vi "test harness_FXP_A_times_x_iterate.vi"() -> ()   [LabVIEW 2017, in "FXP_observer_TestCase.lvclass"]
uses:
  FXP_observer_TestCase.lvclass
  fpga_VIs/fixed-point/typeDefs/x_vec_scalar.ctl
  <vilib>/rvi/DesktopExecutionNode/Execution/niFpgaDEN_Execute.vi
  <vilib>/rvi/DesktopExecutionNode/DesktopExecutionNode.xnode
panel:
  out "X_vec":T1[](array[typedef])
  out "xk_1_1":fxp<+/-,32,6>[](array[numeric])
  out "A*x":fxp<+/-,32,13>[](array[numeric])
  out "y(exp)":fxp<+/-,64,17>
  out "A*x (expected)":fxp<+/-,64,12>[](array[numeric])
  out "Waveform Graph":dbl[](graph)
  out "Y":fxp<+/-,32,6>[](array[numeric])
  in  "NumIter":i32
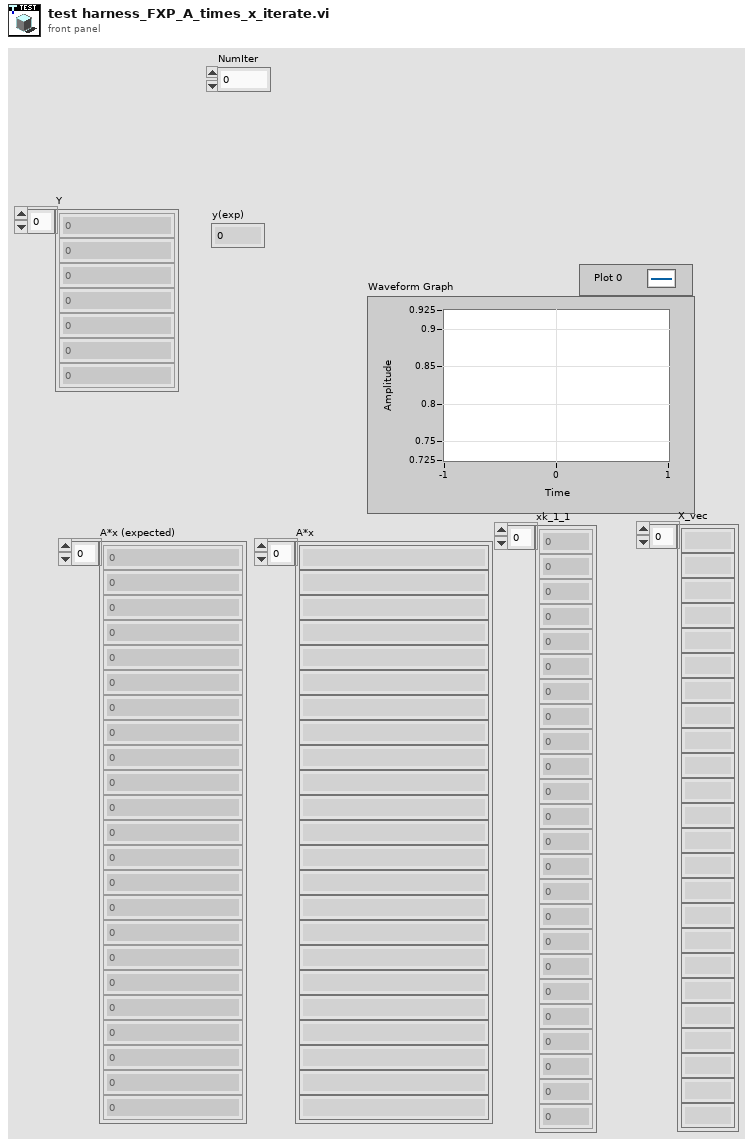
[diagram p1: front panel]
types:
  T1 = typedef "x_vec_scalar.ctl" = fxp<+/-,32,6>
  T2 = typedef "UT_matrix_data.ctl" = cluster{"Bz":T3[], "Ldist":T4[], "Kz":T5[], "Nx":T6[], "Ax_col":T7[], "X_vec":T1[], "Cz":T8[]}
  T3 = typedef "Bz_vec_scalar.ctl" = fxp<+/-,32,3>
  T4 = typedef "Lz_vec_scalar.ctl" = fxp<+/-,32,3>
  T5 = typedef "Kz_vec_scalar.ctl" = fxp<+/-,32,10>
  T6 = typedef "Nx_vec_scalar.ctl" = fxp<+/-,32,2>
  T7 = typedef "Az_vec_scalar.ctl" = fxp<+/-,32,7>
  T8 = typedef "Cz_vec_scalar.ctl" = fxp<+/-,32,4>
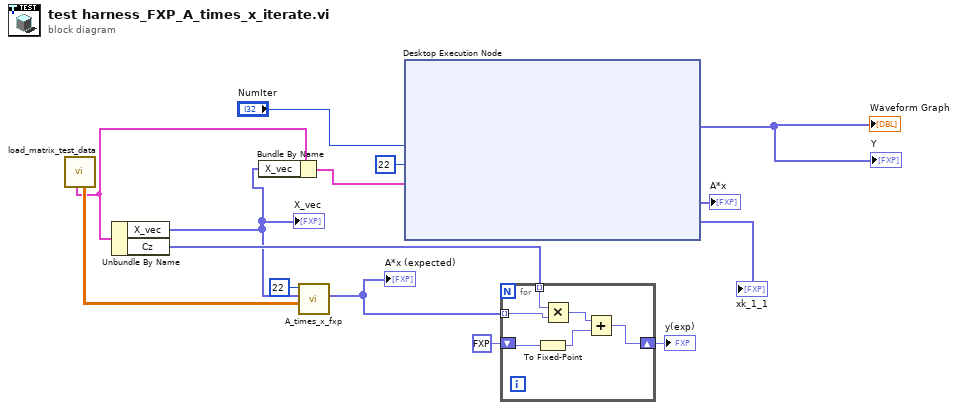
[diagram p0: block diagram]
diagram:
  n1 = call "load_matrix_test_data.vi"() -> ("A_mat"=w11:dbl[][], "output cluster"=w3:T2)  [unwired: 5 in, 5 out]
  n2 = Unbundle By Name(w3) -> ("X_vec"=w1:T1[], "Cz"=w9:T8[])
  "X_vec" <- w1
  n3 = Bundle By Name(cluster=w3, "X_vec"=w1) -> (w2:T2)
  n4 = call "A_times_x_fxp.vi"("Az_mat in"=w11, "x_k"=w1, "NS"=u8 22) -> ("A*x"=w10:fxp<+/-,64,12>[])  [unwired: 7 in, 1 out]
  "A*x (expected)" <- w10
  n5 = xnode "Desktop Execution Node"("NumIter"="NumIter", "NS + 1"=u8 22, "matrix data"=w2) -> ("Y"=→"Y" →"Waveform Graph":fxp<+/-,32,6>[], "A*x"=→"A*x":fxp<+/-,32,13>[], "xk_1_1"=→"xk_1_1":fxp<+/-,32,6>[])  [unwired: 1 in, 1 out]
  n6 = for {
    tunnel: w10 -> [w19] mode=indexing
    tunnel: w9 -> [w20] mode=indexing
    shift-right: [w17] -> w7
    shift-left: fxp<+/-,64,17> 0.0 -> [w15]
    n7 = To Fixed-Point(number=w15) -> (fixed-point=w16:fxp<+/-,64,13>)  [unwired: 1 in]
    n8 = Multiply(x=w20, y=w19) -> (x*y=w18:fxp<+/-,64,16>)
    n9 = Add(x=w18, y=w16) -> (x+y=w17:fxp<+/-,64,17>)
  }
  "y(exp)" <- w7
